vi "SetBoolean.vi"(1 "Boolean":bool, 2 "Attribute":string) -> (0 "Error":bool)   [LabVIEW 2014]
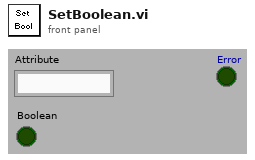
[diagram p1: front panel]
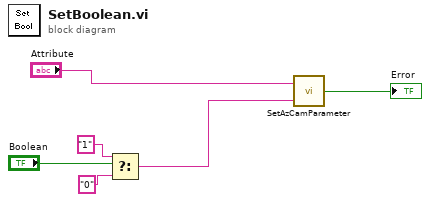
[diagram p0: block diagram]
diagram:
  n1 = Select(t="1", s="Boolean", f="0") -> (s? t:f=w2:string)
  n2 = call "SetAzCamParameter.vi"("Value"=w2, "Parameter"="Attribute") -> ("Error"=→"Error":bool)
